vi "3d_Select_Vertices.vi"(9 "Y index":i32, 10 "X index":i32, 11 "GRID Array":dbl[][](array[numeric])) -> (0 "V4":dbl, 1 "V3":dbl, 2 "V2":dbl, 3 "V1":dbl)   [LabVIEW 2016]
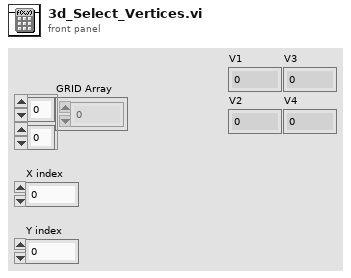
[diagram p1: front panel]
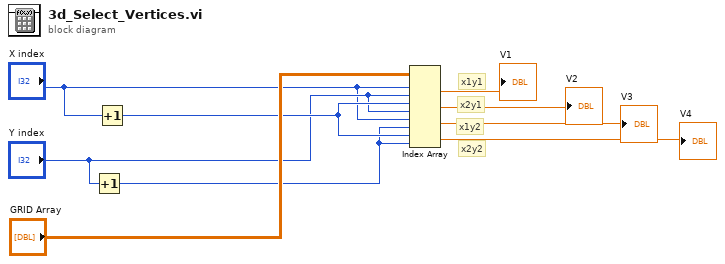
[diagram p0: block diagram]
diagram:
  # "x2y2"
  # "x1y2"
  # "x2y1"
  # "x1y1"
  n1 = Increment(x="Y index") -> (x+1=w1:i32)
  n2 = Increment(x="X index") -> (x+1=w4:i32)
  n3 = Index Array(array="GRID Array", index (row) #1="X index", index (col) #1="Y index", index (row) #2=w4, index (col) #2="Y index", index (row) #3="X index", index (col) #3=w1, index (row) #4=w4, index (col) #4=w1) -> (element #1=→"V1":dbl, element #2=→"V2":dbl, element #3=→"V3":dbl, element #4=→"V4":dbl)
